vi "11.有限点采样.vi"() -> ()   [LabVIEW 2019]
uses:
  <vilib>/rvi/Emulation/niFpgaGetClockAttributes.vi
  <vilib>/rvi/Emulation/niFpgaSctlEmulationGetInTimedLoop.vi
  <vilib>/rvi/Emulation/niFpgaEmulationReportErrorSimple.vi
  <vilib>/rvi/eio/common/nirviEmuTemplateMethod_errors.vi
  <vilib>/rvi/Emulation/niFpgaCriticalErrorInLSC.vi
  <vilib>/eio/EIONode/EIONode.xnode
panel:
  in  "采样点数":i32=300000
  in  "ConnectorA/AO0":sgl(slide) scale=1.0..5.0
  in  "Count(uSec)":u16=100 caption="计数器(uSec)"
  out "ConnectorA/AI0":fxp<+/-,24,5>
  in  "阈值":fxp<+/-,24,5>=3.0
  out "布尔":bool
  in  "Count(uSec) 2":u16=10 caption="计数器(uSec)"
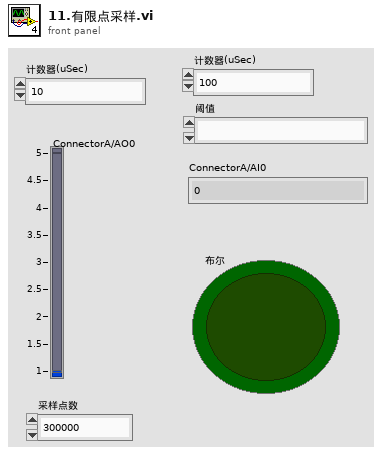
[diagram p1: front panel]
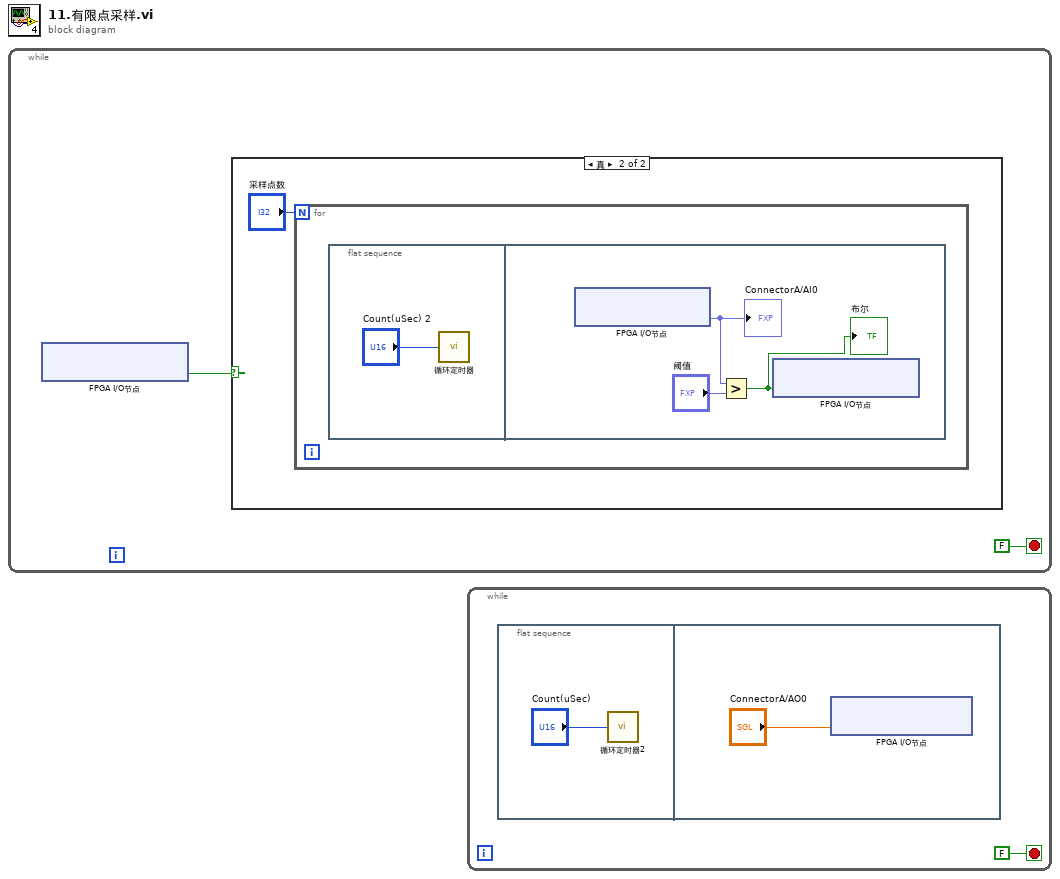
[diagram p0: block diagram]
diagram:
  n1 = while {
    stop <- FALSE stop-if-true
    n2 = xnode "FPGA I/O节点"() -> ("ConnectorA/DIO1"=w1:bool)  [unwired: 1 in, 1 out]
    n3 = case shown="真" w1 {
      frame False {
      }
      frame True {
        n4 = for {
          N: "采样点数" -> [_]
          n5 = flat-sequence {
            frame #0 {
              n6 = call "循环定时器"("Count(uSec)"="Count(uSec) 2") -> ()  [unwired: 1 out]
            }
            frame #1 {
              n7 = xnode "FPGA I/O节点"() -> ("ConnectorA/AI0"=w7:fxp<+/-,24,5>)  [unwired: 1 in, 1 out]
              "ConnectorA/AI0" <- w7
              n8 = Greater?(x=w7, y="阈值") -> (0:w5:bool)
              "布尔" <- w5
              n9 = xnode "FPGA I/O节点"("ConnectorA/DIO0"=w5) -> ()  [unwired: 1 in, 1 out]
            }
          }
        }
      }
    }
  }
  n10 = while {
    stop <- FALSE stop-if-true
    n11 = flat-sequence {
      frame #0 {
        n12 = call "循环定时器2"("Count(uSec)"="Count(uSec)") -> ()  [unwired: 1 out]
      }
      frame #1 {
        n13 = xnode "FPGA I/O节点"("ConnectorA/AO0"="ConnectorA/AO0") -> ()  [unwired: 1 in, 1 out]
      }
    }
  }
